vi "Value To Audio File Refnum.vi"(11 "Refnum Value":i32) -> (3 "Audio File Refnum":T1)   [LabVIEW 2020, in "G-Audio.lvlib"]
uses:
  G-Audio.lvlib
  Controls/Audio File Refnum.ctl
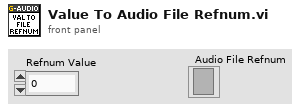
[diagram p1: front panel]
types:
  T1 = typedef "G-Audio.lvlib/Audio File Refnum.ctl" = refnum<file>
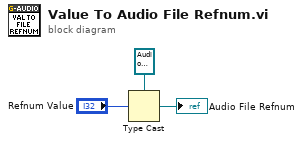
[diagram p0: block diagram]
diagram:
  n1 = Type Cast(type=T1 refnum ("Audio File Refnum"), x="Refnum Value") -> (*(type *) &x=→"Audio File Refnum":T1)
